vi "Extract Angles.vi"(8 "Induced disturbance":dbl format="%#_13g", 11 "String in":string) -> (1 "Output":T1)   [LabVIEW 2016]
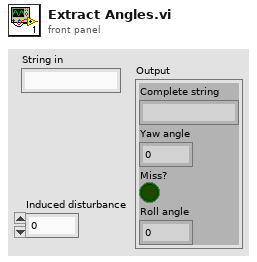
[diagram p1: front panel]
types:
  T1 = cluster{"Complete string":string, "Yaw angle":dbl, "Miss?":bool, "Roll angle":dbl}
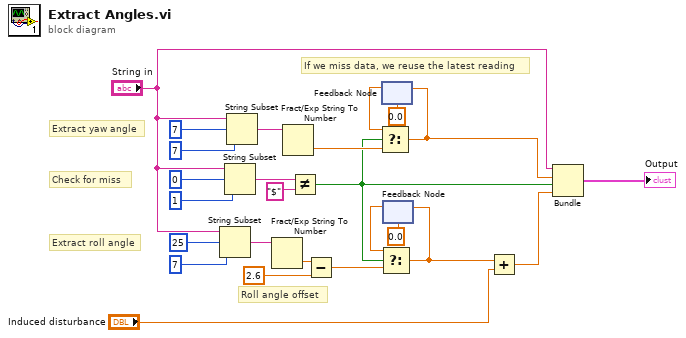
[diagram p0: block diagram]
diagram:
  # "If we miss data, we reuse the latest reading"
  # "Check for miss"
  # "Extract yaw angle"
  # "Extract roll angle"
  # "Roll angle offset"
  n1 = String Subset(string="String in", offset (0)=25, length (rest)=7 ("length (rest)")) -> (substring=w16:string)
  n2 = String Subset(string="String in", offset (0)=0 ("length (rest)"), length (rest)=1 ("length (rest)")) -> (substring=w18:string)
  n3 = String Subset(string="String in", offset (0)=7, length (rest)=7 ("length (rest)")) -> (substring=w23:string)
  n4 = Fract/Exp String To Number(string=w16) -> (number=w21:dbl)  [unwired: 3 in, 1 out]
  n5 = Fract/Exp String To Number(string=w23) -> (number=w13:dbl)  [unwired: 3 in, 1 out]
  n6 = Not Equal?(x=w18, y="$") -> (x != y?=w6:bool)
  n7 = Subtract(x=w21, y=2.6) -> (x-y=w9:dbl)
  n8 = feedback #1(0.0) -> (w12:dbl)
  n9 = Select(t=w12, s=w6, f=w13) -> (s? t:f=w10:dbl)
  n10 = feedback-in #1(w10) -> ()
  n11 = feedback #2(0.0) -> (w8:dbl)
  n12 = Select(t=w8, s=w6, f=w9) -> (s? t:f=w4:dbl)
  n13 = feedback-in #2(w4) -> ()
  n14 = Add(x=w4, y="Induced disturbance") -> (x+y=w3:dbl)
  n15 = Bundle("String in"="String in", w10, w6, w3) -> (→"Output":cluster{"String in":string, dbl, bool, dbl})  [unwired: 1 in]
